vi "Get Axis.vi"(8 "error in (no error)":errorcluster, 11 "Synapse CCD.lvclass In":refnum<class "Synapse CCD.lvclass">) -> (0 "error out":errorcluster, 2 "Array of Wavelengths":dbl[](array[numeric]), 3 "Synapse CCD.lvclass Out":refnum<class "Synapse CCD.lvclass">)   [LabVIEW 2015, in "Synapse CCD.lvclass"]
doc: "Reads the linearized wavelengths from last Data Acquisition, returns as Array of DBLs."
uses:
  Synapse CCD.lvclass
  Synapse CCD.lvclass/Synapse CCD.ctl
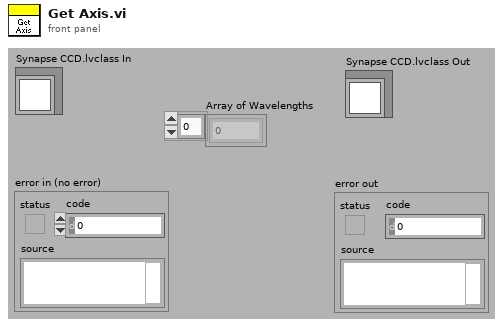
[diagram p1: front panel]
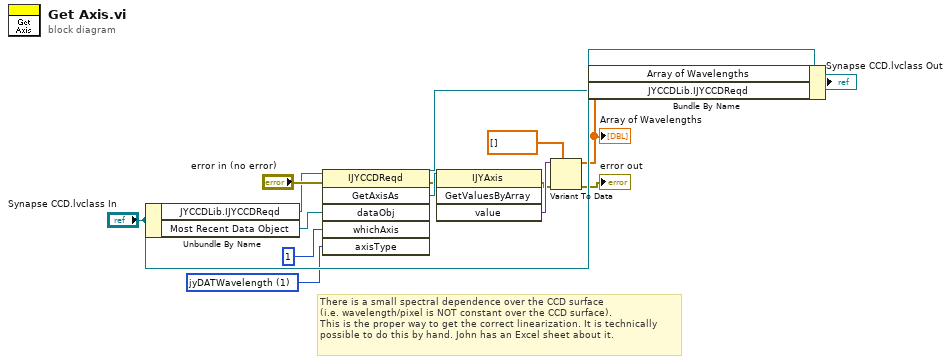
[diagram p0: block diagram]
diagram:
  w7 = 1 items=["jyDATUndefined", "jyDATWavelength", "jyDATPixel", "jyDATMillimeters", "jyDATMicrometers"] ("axisType")
  # "There is a small spectral dependence over the CCD surface\n(i.e. wavelength/pixel is NOT constant over the CCD surface).\nThis is the proper way to get the correct linearization. It is technically\npossible to do this by hand. John has an Excel sheet about it."
  n1 = Unbundle By Name("Synapse CCD.lvclass In") -> ("JYCCDLib.IJYCCDReqd"=w11:refnum<k7>, "Most Recent Data Object"=w15:refnum<k7>)
  n2 = invoke class="IJYCCDReqd" method="GetAxisAs"(reference=w11, error in="error in (no error)", "dataObj"=w15, "whichAxis"=1, "axisType"=w7) -> (reference out=w8:refnum<k7>, error out=w4:errorcluster, "GetAxisAs"=w5:refnum<k7>)  [unwired: 1 in, 3 out]
  n3 = invoke class="IJYAxis" method="GetValuesByArray"(reference=w5, error in=w4) -> (error out=w1:errorcluster, "value"=w3:variant)  [unwired: 2 in, 2 out]
  n4 = Variant To Data(error in=w1, type=dbl[] [], Variant=w3) -> (data=w9:dbl[], error out=→"error out":errorcluster)
  "Array of Wavelengths" <- w9
  n5 = Bundle By Name(cluster="Synapse CCD.lvclass In", "Array of Wavelengths"=w9, "JYCCDLib.IJYCCDReqd"=w8) -> (→"Synapse CCD.lvclass Out":refnum<class "Synapse CCD.lvclass">)
